vi "SwerveAssistStrafe.vi"(1 "In Deadband":bool, 2 "Joystick X":dbl, 3 "Joystick Y":dbl, 7 "Strafe PID":T2={"Kp"=0.1, "Ki"=0.1, "Kd"=0.1, "N-Diff"=10, "N-Int"=20, "Int Error Window"=0.5, "Max Ouput"=1.0, "Min Output"=-1.0, "Square Derivative"=FALSE, "N-Prop"=1} {"N-Prop" min=1; "Int Error Window" min=0.0; "N-Int" min=2; "N-Diff" min=2; "Kd" min=0.0; "Ki" min=0.0; "Kp" min=0.0}, 8 "Locked Y (in)":dbl format="%#_13g", 10 "Orientation Mode":enum16{"Robot-Oriented", "Field-Oriented"}(ring)) -> (14 "Strafe PID Plot":T1, 15 "In Deadband":bool, 16 "Assisted X":dbl, 17 "Assisted Y":dbl, 19 "Strafe Assist On":bool)   [LabVIEW 2020]
doc: "Runs a PID controller to maintain the robot's postion relative to a vector parallel to the field's x-axis. If no goal y position is given, the driver commands are passed through unaltered."
uses:
  af15fe63-c48f-490d-b061-1826781410b4.vi
  GlobalPoseAndTargeting.vi
  GlobalDriverStationCommands.vi
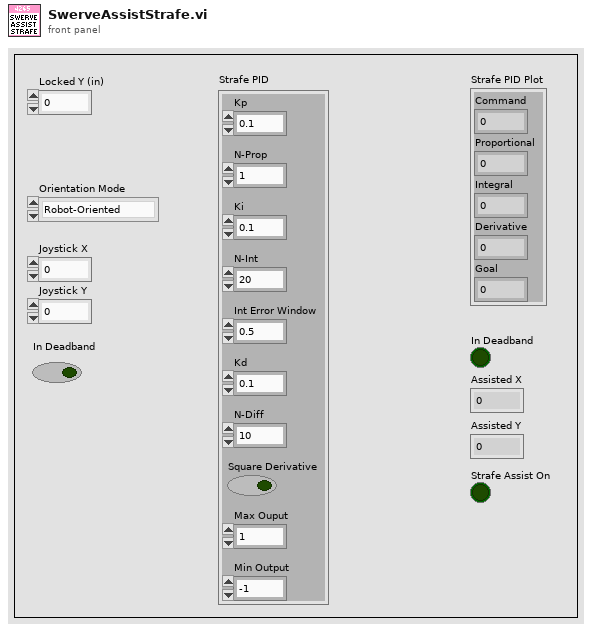
[diagram p1: front panel]
types:
  T1 = cluster{"Command":dbl, "Proportional":dbl, "Integral":dbl, "Derivative":dbl, "Goal":dbl}
  T2 = cluster{"Kp":dbl, "Ki":dbl, "Kd":dbl, "N-Diff":i32, "N-Int":i32, "Int Error Window":dbl, "Max Ouput":dbl, "Min Output":dbl, "Square Derivative":bool, "N-Prop":i32}
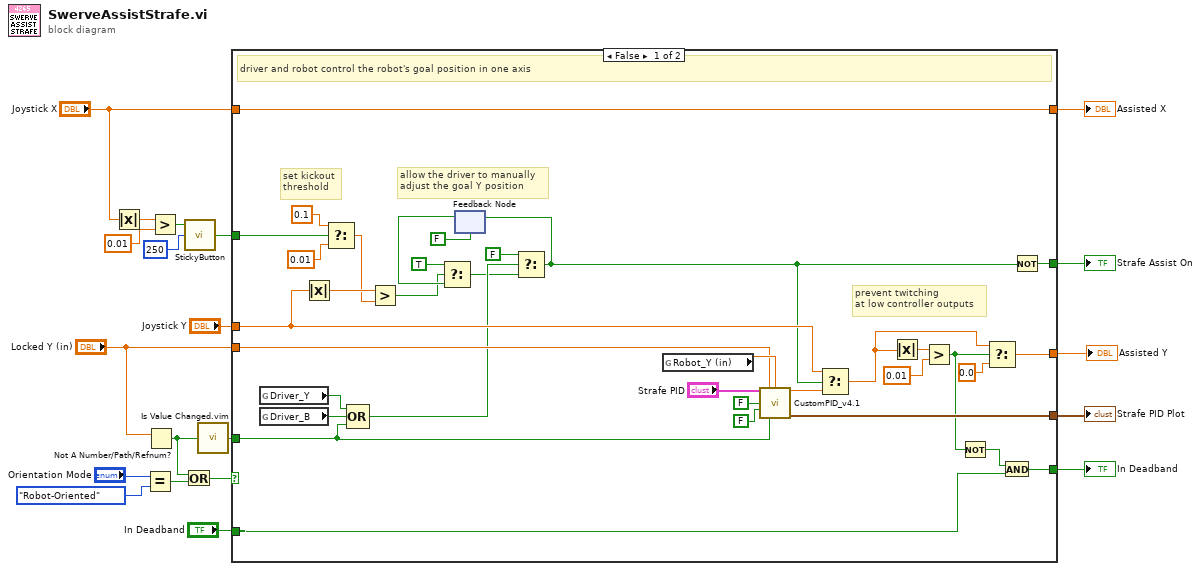
[diagram p0: block diagram]
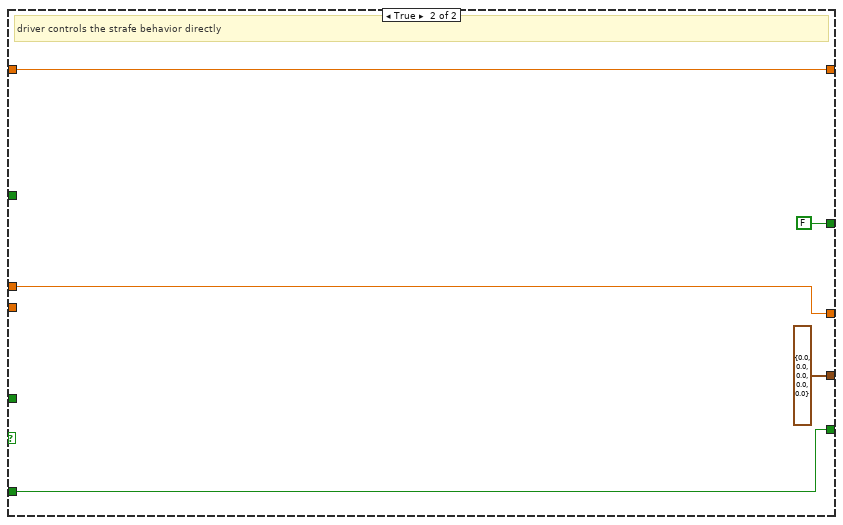
[diagram p2: hidden frame]
diagram:
  n1 = Absolute Value(x="Joystick X") -> (abs(x)=w1:dbl)
  n2 = Equal?(x="Orientation Mode", y=enum16{"Robot-Oriented", "Field-Oriented"}."Robot-Oriented") -> (x = y?=w8:bool)
  n3 = Not A Number/Path/Refnum?(number/path/refnum="Locked Y (in)") -> (NaN/Path/Refnum?=w9:bool)
  n4 = Greater?(x=w1, y=0.01) -> (0:w4:bool)
  n5 = Or(x=w9, y=w8) -> (x .or. y?=w10:bool)
  n6 = call "StickyButton.vi"("Time threshold (ms)"=u32 250, "Button Input"=w4) -> ("Sticky Button"=w3:bool)  [unwired: 1 in]
  n7 = call "Is Value Changed.vim"("value"=w9) -> ("changed or first call?"=w20:bool)
  n8 = case shown="False" w10 {
    tunnel: "Locked Y (in)" -> [w35 _]
    tunnel: [w53 T1 {"Command"=0.0, "Proportional"=0.0, "Integral"=0.0, "Derivative"=0.0, "Goal"=0.0} ("Controller Summary")] -> w16
    tunnel: [w49 w56] -> w14
    tunnel: [w47 w58] -> w17
    tunnel: w20 -> [w38 _]
    tunnel: "In Deadband" -> [w46 w58]
    tunnel: [w23 FALSE] -> w15
    tunnel: "Joystick Y" -> [w41 w56]
    tunnel: "Joystick X" -> [w28 w60]
    tunnel: [w28 w60] -> w13
    tunnel: w3 -> [w22 _]
    frame False {
      # "set kickout\nthreshold"
      # "allow the driver to manually\nadjust the goal Y position"
      # "prevent twitching\nat low controller outputs"
      # "driver and robot control the robot's goal position in one axis"
      n9 = global read "GlobalDriverStationCommands.vi" "Driver_Y"() -> (w21:bool)
      n10 = global read "GlobalDriverStationCommands.vi" "Driver_B"() -> (w39:bool)
      n11 = Absolute Value(x=w41) -> (abs(x)=w37:dbl)
      n12 = Select(t=0.1 ("y"), s=w22, f=0.01) -> (s? t:f=w27:dbl)
      n13 = Compound Arithmetic op=OR(w21, w39, w38) -> (w34:bool)
      n14 = Greater?(x=w37, y=w27) -> (0:w31:bool)
      n15 = feedback #1(FALSE) -> (w32:bool)
      n16 = Select(t=TRUE, s=w31, f=w32) -> (s? t:f=w33:bool)
      n17 = Select(t=FALSE, s=w34, f=w33) -> (s? t:f=w24:bool)
      n18 = feedback-in #1(w24) -> ()
      n19 = global read "GlobalPoseAndTargeting.vi" "Robot_Y (in)"() -> (w40:dbl)
      n20 = call "CustomPID_v4.1.vi"("PID Tuning Parameters"="Strafe PID", "Goal"=w35, "Process Variable"=w40, "Reset on Goal Change ?"=FALSE, "Use Custom Error Calculation ?"=FALSE, "Reinit"=w38) -> ("Command"=w43:dbl, "Controller Summary"=w53:T1)  [unwired: 6 in, 2 out]
      n21 = Select(t=w41, s=w24, f=w43) -> (s? t:f=w42:dbl)
      n22 = Absolute Value(x=w42) -> (abs(x)=w52:dbl)
      n23 = Greater?(x=w52, y=0.01) -> (0:w44:bool)
      n24 = Not(x=w44) -> (.not. x?=w45:bool)
      n25 = Select(t=w42, s=w44, f=0.0 ("t")) -> (s? t:f=w49:dbl)
      n26 = And(x=w45, y=w46) -> (x .and. y?=w47:bool)
      n27 = Not(x=w24) -> (.not. x?=w23:bool)
    }
    frame True {
      # "driver controls the strafe behavior directly"
    }
  }
  "Assisted X" <- w13
  "Strafe Assist On" <- w15
  "Strafe PID Plot" <- w16
  "In Deadband" <- w17
  "Assisted Y" <- w14
